vi "log_file_test.vi"() -> ()   [LabVIEW 2013]
uses:
  global_log_file.vi
panel:
  in  "Tab Control":T1(tab)=enum."Standard Motor Operation"
  out "Created New Semaphor":bool
  in  "error in (no error)":errorcluster
  out "error out":errorcluster
  in  "Test-String":string
  in  "TEST":bool
  out "Log File 2":string
  in  "Delete Log File 2":bool
  in  "Delete Log File":bool
  out "Log File":string
  in  "stop":bool
  # "(leave out # and \\r)"
  # "(\"?\" means Command is invalid)"
  # "(in Hz)"
  # "(in Hz)"
  # "(in Hz/ms)"
  # "(in Hz/ms)"
  # "[1-32]"
  # "STEPS"
  # "Standard Profile Parameters for Operation of Motors (V_Start, V_Stop, Ramp, Break, etc.)\nfor this Tab can be manipulated in the Code (Event-Structure Frame 20)."
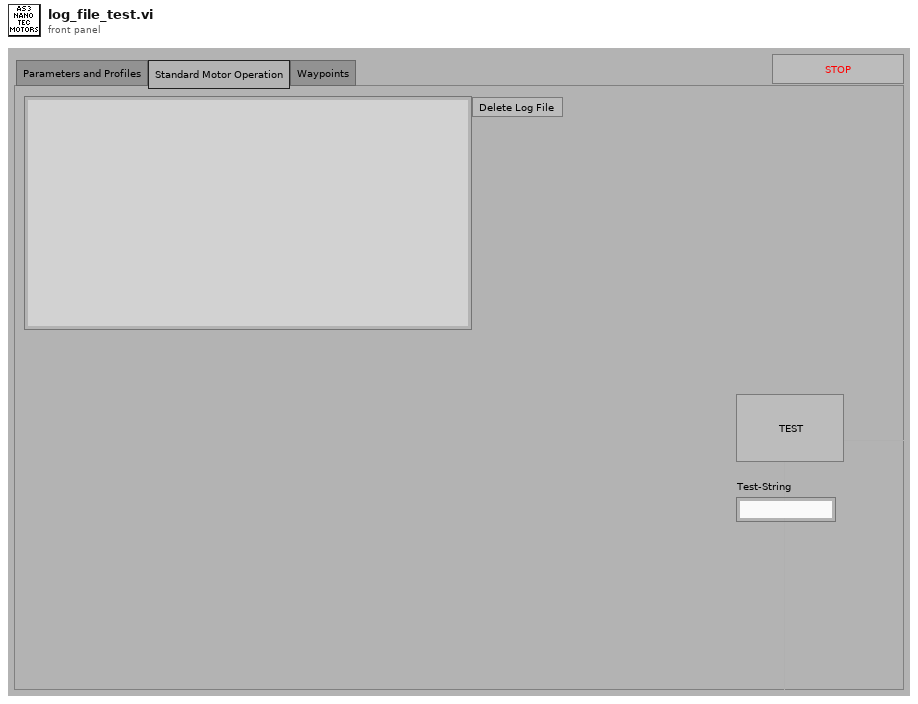
[diagram p1: front panel]
types:
  T1 = enum32{"Parameters and Profiles", "Standard Motor Operation", "Waypoints"}
  T2 = enum16{"open", "replace", "create", "open or create", "replace or create", "replace or create with confirmation"}
  T3 = typedef "Semaphore RefNum" = refnum<k1>
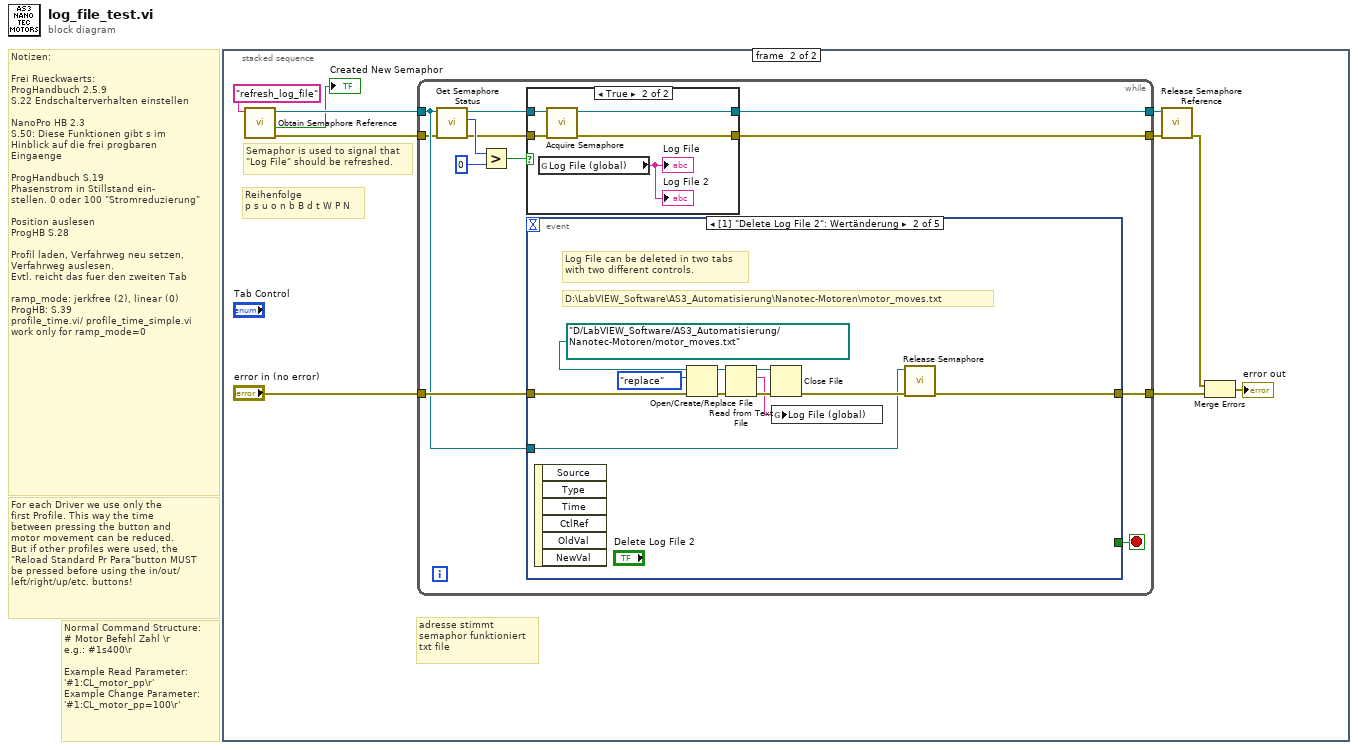
[diagram p0: block diagram]
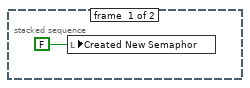
[diagram p2: hidden frame]
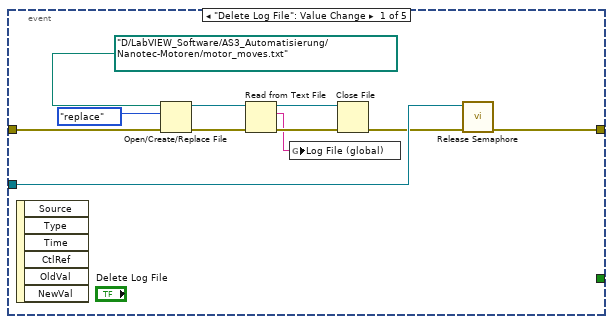
[diagram p4: hidden frame]
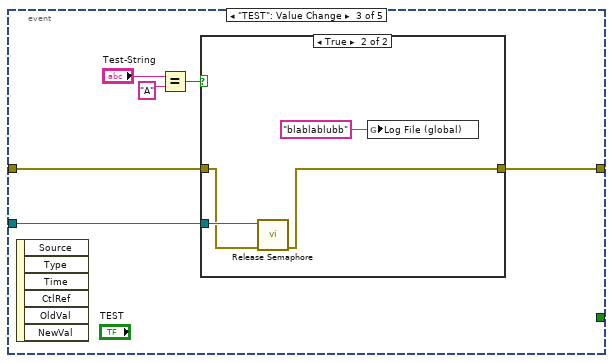
[diagram p5: hidden frame]
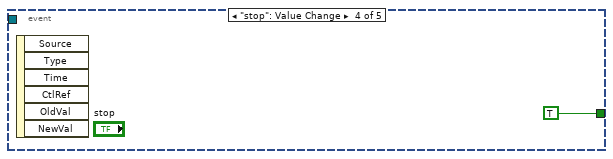
[diagram p7: hidden frame]
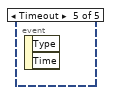
[diagram p8: hidden frame]
diagram:
  # "For each Driver we use only the\nfirst Profile. This way the time\nbetween pressing the button and\nmotor movement can be reduced.\nBut if other profiles were used, the\n\"Reload Standard Pr Para\"button MUST\nbe pressed before using the in/out/\nleft/right/up/etc. buttons!"
  # "Normal Command Structure:\n# Motor Befehl Zahl \\r\ne.g.: #1s400\\r\n\nExample Read Parameter:\n'#1:CL_motor_pp\\r'\nExample Change Parameter:\n'#1:CL_motor_pp=100\\r'"
  # "Notizen:\n\nFrei Rueckwaerts:\nProgHandbuch 2.5.9\nS.22 Endschalterverhalten einstellen\n\nNanoPro HB 2.3 \nS.50: Diese Funktionen gibt s im \nHinblick auf die frei progbaren \nEingaenge\n\nProgHandbuch S.19\nPhasenstrom in Stillstand ein-\nstellen. 0 oder 100 \"Stromreduzierung\"\n\nPosition auslesen\nProgHB S.28\n\nProfil laden, Verfahrweg neu setzen,\nVerfahrweg auslesen.\nEvtl. reicht das fuer den zweiten Tab\n\nramp_mode: jerkfree (2), linear (0) \nProgHB: S.39\nprofile_time.vi/ profile_time_simple.vi\nwork only for ramp_mode=0"
  n1 = stacked-sequence {
    frame #0 {
      n2 = local write "Created New Semaphor"(FALSE) -> ()
    }
    frame #1 {
      # "adresse stimmt\nsemaphor funktioniert\ntxt file"
      # "Reihenfolge\np s u o n b B d t W P N"
      # "Semaphor is used to signal that\n\"Log File\" should be refreshed."
      n3 = call <vilib>:"Obtain Semaphore Reference.vi"("name (unnamed)"="refresh_log_file") -> ("error out"=w8:errorcluster, "created new"=→"Created New Semaphor":bool, "semaphore"=w10:T3)  [unwired: 4 in]
      n4 = while {
        tunnel: "error in (no error)" -> [w23]
        tunnel: [w12] -> w2
        tunnel: w10 -> [w17]
        tunnel: [w18] -> w9
        tunnel: w8 -> [w16]
        tunnel: [w14] -> w7
        stop <- w13 stop-if-true
        n5 = call <vilib>:"Get Semaphore Status.vi"("error in (no error)"=w16, "semaphore"=w17) -> ("error out"=w15:errorcluster, "# available"=w22:i32, "semaphore out"=w19:T3)  [unwired: 4 in, 3 out]
        n6 = Greater?(x=w22, y=0) -> (0:w20:bool)
        n7 = case shown="True" w20 {
          tunnel: w19 -> [w25 w30]
          tunnel: [w25 w29] -> w18
          tunnel: w15 -> [w24 w28]
          tunnel: [w24 w27] -> w14
          frame False {
          }
          frame True {
            n8 = global read "global_log_file.vi" "Log File (global)"() -> (→"Log File" →"Log File 2":string)
            n9 = call <vilib>:"Acquire Semaphore.vi"("error in (no error)"=w28, "semaphore"=w30) -> ("error out"=w27:errorcluster, "semaphore out"=w29:T3)  [unwired: 3 in, 1 out]
          }
        }
        n10 = event shown="[1] \"Delete Log File 2\": Wertänderung" {
          selector: _ -> [_ _ _ _ _]
          dyn-events: _ -> [_ _ _ _ _]
          timeout: _ -> [_ _ _ _ _]
          tunnel: w23 -> [w38 w45 w54 _ _]
          tunnel: [w39 w43 w53 _ _] -> w12
          tunnel: w17 -> [w40 w44 w55 _ _]
          tunnel: [_ _ _ TRUE _] -> w13
          event "Delete Log File": Value Change {
            n11 = event-data() -> ()  [unwired: 1 in, 6 out]
            n12 = Open/Create/Replace File(file path (use dialog)=path "D:/LabVIEW_Software/AS3_Automatisierung/Nanotec-Motoren/motor_moves.txt", error in=w38, operation (0:open)=T2."replace") -> (refnum out=w34:refnum<file>, error out=w36:errorcluster)  [unwired: 3 in, 1 out]
            n13 = Read from Text File(file (use dialog)=w34, error in=w36) -> (refnum out=w33:refnum<file>, text=w32:string, error out=w37:errorcluster)  [unwired: 2 in, 1 out]
            n14 = global write "global_log_file.vi" "Log File (global)"(w32) -> ()
            n15 = Close File(refnum=w33, error in=w37) -> (error out=w35:errorcluster)  [unwired: 1 out]
            n16 = call <vilib>:"Release Semaphore.vi"("error in (no error)"=w35, "semaphore"=w40) -> ("error out"=w39:errorcluster)  [unwired: 4 in, 1 out]
          }
          event "Delete Log File 2": Value Change {
            # "D:\\LabVIEW_Software\\AS3_Automatisierung\\Nanotec-Motoren\\motor_moves.txt"
            # "Log File can be deleted in two tabs\nwith two different controls."
            n17 = event-data() -> ()  [unwired: 1 in, 6 out]
            n18 = Open/Create/Replace File(file path (use dialog)=path "D:/LabVIEW_Software/AS3_Automatisierung/Nanotec-Motoren/motor_moves.txt", error in=w45, operation (0:open)=T2."replace") -> (refnum out=w48:refnum<file>, error out=w50:errorcluster)  [unwired: 3 in, 1 out]
            n19 = Read from Text File(file (use dialog)=w48, error in=w50) -> (refnum out=w47:refnum<file>, text=w46:string, error out=w51:errorcluster)  [unwired: 2 in, 1 out]
            n20 = Close File(refnum=w47, error in=w51) -> (error out=w49:errorcluster)  [unwired: 1 out]
            n21 = global write "global_log_file.vi" "Log File (global)"(w46) -> ()
            n22 = call <vilib>:"Release Semaphore.vi"("error in (no error)"=w49, "semaphore"=w44) -> ("error out"=w43:errorcluster)  [unwired: 4 in, 1 out]
          }
          event "TEST": Value Change {
            n23 = event-data() -> ()  [unwired: 1 in, 6 out]
            n24 = Equal?(x="Test-String", y="A") -> (x = y?=w56:bool)
            n25 = case shown="True" w56 {
              tunnel: w55 -> [_ w63]
              tunnel: w54 -> [w59 w62]
              tunnel: [w59 w61] -> w53
              frame False {
              }
              frame True {
                n26 = call <vilib>:"Release Semaphore.vi"("error in (no error)"=w62, "semaphore"=w63) -> ("error out"=w61:errorcluster)  [unwired: 4 in, 1 out]
                n27 = global write "global_log_file.vi" "Log File (global)"("blablablubb") -> ()
              }
            }
          }
          event "stop": Value Change {
            n28 = event-data() -> ()  [unwired: 1 in, 6 out]
          }
          event Timeout {
            n29 = event-data() -> ()  [unwired: 1 in, 2 out]
          }
        }
      }
      n30 = call <vilib>:"Release Semaphore Reference.vi"("error in (no error)"=w7, "semaphore"=w9) -> ("error out"=w5:errorcluster)  [unwired: 8 in, 1 out]
      n31 = Merge Errors(w5, w2) -> (→"error out":errorcluster)
    }
  }
